vi "Create Device Reference.vi"(8 "error in (no error)":errorcluster, 11 "SerialNumber":string="97000001") -> (0 "error out":errorcluster, 2 "Device":refnum<k24>, 3 "KCubeInertialMotorControl out":refnum<k24>, 5 "CreateDevice Result":bool)   [LabVIEW 2017]
uses:
  D:/upwork/Laser Measurement Tool/Laser/tests/KIM101/Thorlabs.MotionControl.Controls.dll
  Thorlabs.MotionControl.Controls.dll
  D:/upwork/Laser Measurement Tool/Laser/tests/KIM101/Thorlabs.MotionControl.KCube.InertialMotorCLI.dll
  Thorlabs.MotionControl.KCube.InertialMotorCLI.dll
panel:
  in  "KCubeInertialMotorControl":refnum<k24>(container)
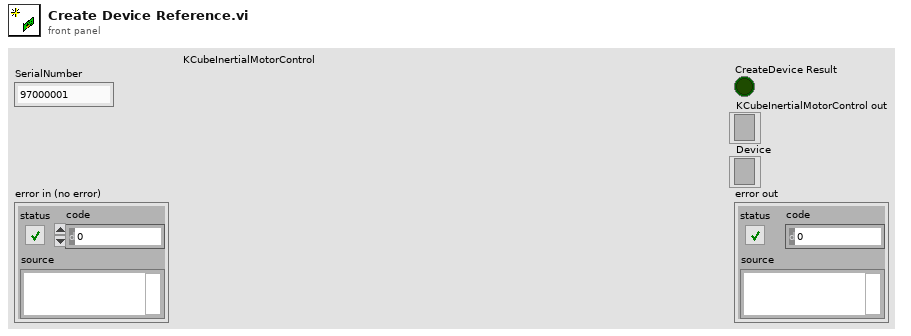
[diagram p1: front panel]
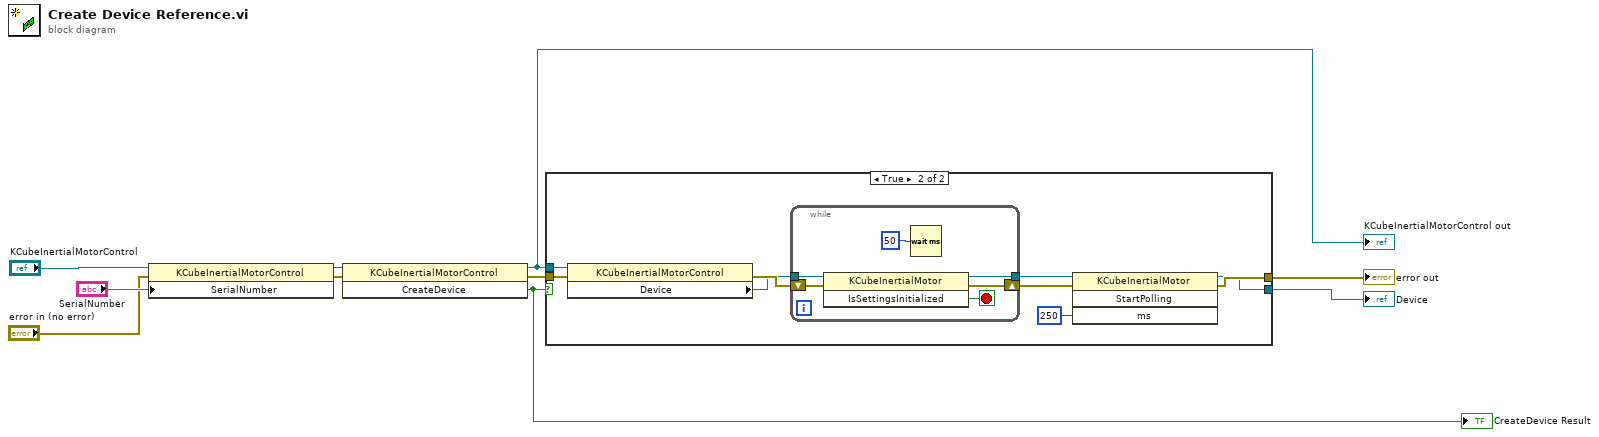
[diagram p0: block diagram]
diagram:
  n1 = property class="KCubeInertialMotorControl"(reference="KCubeInertialMotorControl", error in="error in (no error)", "SerialNumber"="SerialNumber") -> (reference out=w8:refnum<k24>, error out=w7:errorcluster)
  n2 = invoke class="KCubeInertialMotorControl" method="CreateDevice"(reference=w8, error in=w7) -> (reference out=w3:refnum<k24>, error out=w5:errorcluster, "CreateDevice"=w6:bool)  [unwired: 1 in]
  "CreateDevice Result" <- w6
  "KCubeInertialMotorControl out" <- w3
  n3 = case shown="True" w6 {
    tunnel: w3 -> [_ w19]
    tunnel: w5 -> [w11 w20]
    tunnel: [_ w12] -> w1
    tunnel: [w11 w13] -> w4
    frame False {
    }
    frame True {
      n4 = property class="KCubeInertialMotorControl"(reference=w19, error in=w20) -> (error out=w15:errorcluster, "Device"=w14:refnum<k24>)  [unwired: 1 out]
      n5 = while {
        tunnel: [w25] -> w18
        tunnel: w14 -> [w21]
        shift-right: [w22] -> w16
        shift-left: w15 -> [w23]
        stop <- w26 stop-if-true
        n6 = invoke class="KCubeInertialMotor" method="IsSettingsInitialized"(reference=w21, error in=w23) -> (reference out=w25:refnum<k24>, error out=w22:errorcluster, "IsSettingsInitialized"=w26:bool)  [unwired: 1 in]
        n7 = Wait (ms)(milliseconds to wait=u32 50) -> ()  [unwired: 1 out]
      }
      n8 = invoke class="KCubeInertialMotor" method="StartPolling"(reference=w18, error in=w16, "ms"=250) -> (reference out=w12:refnum<k24>, error out=w13:errorcluster)  [unwired: 1 in, 2 out]
    }
  }
  "error out" <- w4
  "Device" <- w1
